vi "Energize.vi"(8 "error in (no error)":errorcluster, 11 "CIFTemplatePlugin in":refnum<class "TemplatePlugin.lvclass">) -> (0 "error out":errorcluster, 3 "CIFTemplatePlugin out":refnum<class "TemplatePlugin.lvclass">)   [LabVIEW 2021, in "TemplatePlugin.lvlib"]
uses:
  TemplatePlugin.lvlib
  Class/TemplatePlugin.lvclass
  D:/dev/CIF-LVCore/src/CIFCore/Class/CIFCorePlugin.lvclass
  CIF-LVCore/src/CIFCore/Class/CIFCorePlugin.lvclass/CIFCorePlugin.ctl
  <vilib>/Platform/TimedLoop/XDataNode/timing_clust.ctl
  <vilib>/Platform/TimedLoop/XDataNode/nitl_modes.ctl
  <vilib>/Platform/TimedLoop/XDataNode/wakeup.ctl
  Class/TemplatePlugin.lvclass/TemplatePlugin.ctl
  CIF-LVCore/src/Channels/CIFChannelMng/CIFChannelMng.lvclass/CIFChannelMng.ctl
  <vilib>/CIF Foundation/CIF Utilities/Statistics/I64/Stats_I64_CIF_U.lvclass/Stats_I64_CIF_U.ctl
  <vilib>/CIF Foundation/CIF Out of Band Commands/CIFOutOfBand.lvclass/CIFOutOfBand.ctl
  CIF-LVCore/src/CIFCore/OOB/OOB_Rx/CIFCoreOOB_Rx.lvclass/CIFCoreOOB_Rx.ctl
  <vilib>/CIF Foundation/CIF Channels Core/CIFChannels/CIFChannels.lvclass/CIFChannels.ctl
  <vilib>/CIF Foundation/CIF Utilities/Time/System Time/Get System Time.vi
  CIF-LVCore/src/CIFCore/Class/SubVIs/Running State Logic.vi
  Class/Dynamic/Execute.vi
  Class/Dynamic/Housekeeping.vi
  CIF-LVCore/src/CIFCore/Class/SubVIs/Send Core OOB TX.vi
  CIF-LVCore/src/CIFCore/Class/Accessors/Read Energized State.vi
  CIF-LVCore/src/CIFCore/Class/SubVIs/Start Running.vi
  <vilib>/CIF Foundation/CIF Utilities/Time/System Time/LabVIEW Time to TAI Time.vi
  CIF-LVCore/src/CIFCore/Class/Accessors/Timestamps/Write Sleep TS.vi
  CIF-LVCore/src/CIFCore/Class/SubVIs/Sleep.vi
  Class/Dynamic/Logic.vi
  CIF-LVCore/src/CIFCore/Class/Accessors/Write Energized State.vi
  CIF-LVCore/src/CIFCore/Class/Benchmarking/Benchmark Running.vi
  CIF-LVCore/src/CIFCore/Class/SubVIs/Read Core OOB RX.vi
  Class/gRPC/Read gRCP to Main.vi
  Class/gRPC/Send Main to gRPC.vi
  CIF-LVCore/src/CIFCore/Class/SubVIs/OOB/Update Status from Benchmarks.vi
  CIF-LVCore/src/Channels/CIFChannelMng/Core/Send Channel List Update.vi
  <vilib>/CIF Foundation/CIF Utilities/Time/System Time/Sleep Until Future Time.vi
  CIF-LVCore/src/CIFCore/Class/Accessors/Timestamps/Write Execute TS.vi
  <vilib>/Utility/error.llb/Clear Errors.vi
  CIF-LVCore/src/CIFCore/Class/Accessors/Read Sleep Limits (ns).vi
  CIF-LVCore/src/CIFCore/Class/Accessors/Timestamps/Write Target Wake TS.vi
  CIF-LVCore/src/CIFCore/Common/Utilities/Add Error.vi
  CIF-LVCore/src/CIFCore/Class/Accessors/Read Plugin Name.vi
  CIF-LVCore/src/CIFCore/Class/Accessors/Timestamps/Read Running TS.vi
  CIF-LVCore/src/CIFCore/Class/Accessors/Read Running Internal Data.vi
  CIF-LVCore/src/CIFCore/Class/Accessors/Read Timing Override.vi
  CIF-LVCore/src/CIFCore/Class/Accessors/Read Common Config.vi
  CIF-LVCore/src/CIFCore/Class/Channel RW/Read Double.vi
  CIF-LVCore/src/CIFCore/Class/Channel RW/Write Double.vi
  CIF-LVCore/src/CIFCore/Class/Channel RW/Read U64.vi
  CIF-LVCore/src/CIFCore/Class/Channel RW/Write U64.vi
  CIF-LVCore/src/CIFCore/Class/Utilities/Benchmarking/Benchmark Custom 1.vi
  Class/Dynamic/Logic.vi/43ad4f59-20dd-452f-bd87-f699ede29eb7.vi
  Class/Dynamic/Logic.vi/a3a5b85b-e031-4b11-917e-7505e820cabf.vi
  CIF-LVCore/src/CIFCore/Class/Accessors/Monitor/Write Double 1.vi
  CIF-LVCore/src/CIFCore/Class/Accessors/Monitor/Write U64 1.vi
  CIF-LVCore/src/CIFCore/Class/Accessors/Monitor/Write I64 1.vi
  CIF-LVCore/src/CIFCore/Class/Accessors/Monitor/Write I64 2.vi
  CIF-LVCore/src/CIFCore/Class/Accessors/Timestamps/Write Housekeeping TS.vi
  <vilib>/CIF Foundation/CIF Utilities/Statistics/I64/X1 minus X0.vi
  <vilib>/CIF Foundation/CIF Utilities/Statistics/I64/Cyclic.vi
  CIF-LVCore/src/CIFCore/Class/Accessors/Timestamps/Read Execute TS.vi
  CIF-LVCore/src/CIFCore/Class/Accessors/Timestamps/Read Housekeeping TS.vi
  CIF-LVCore/src/CIFCore/Class/Accessors/Timestamps/Read Sleep TS.vi
  CIF-LVCore/src/CIFCore/Class/Accessors/Timestamps/Read Target Wake TS.vi
  CIF-LVCore/src/CIFCore/Class/SubVIs/Refresh Stats.vi
  CIF-LVCore/src/CIFCore/OOB/OOB_Rx/Receive/Read Clock Map.vi
  CIF-LVCore/src/Channels/CIFChannelMng/SubVIs/Connect Channel.vi
  CIF-LVCore/src/CIFCore/OOB/OOB_Rx/Receive/Read Connections.vi
  CIF-LVCore/src/CIFCore/OOB/OOB_Rx/Receive/Read Forces.vi
  CIF-LVCore/src/Channels/CIFChannelMng/SubVIs/Force Channel.vi
  CIF-LVCore/src/Channels/CIFChannelMng/SubVIs/Add FIFO Publisher.vi
  CIF-LVCore/src/CIFCore/OOB/OOB_Rx/Receive/Read Publisher Instance.vi
  CIF-LVCore/src/Channels/CIFChannelMng/Core/Send Publisher Instance Return.vi
  CIF-LVCore/src/Channels/CIFChannelMng/SubVIs/Remove FIFO Publisher.vi
  CIF-LVCore/src/CIFCore/OOB/OOB_Rx/Receive/Check for OOB Commands.vi
  OOB/OOB_Rx/Receive/Read Data.vi
  OOB/OOB_Rx/Receive/Check for OOB Commands.vi
  OOB/OOB_Tx/Send/Update Data.vi
  <vilib>/CIF Foundation/CIF Out of Band Commands/Commit Commands.vi
  CIF-LVCore/src/CIFCore/Class/Accessors/Read Refresh.vi
  <vilib>/CIF Foundation/CIF Utilities/Statistics/I64/Get Stats.vi
  CIF-LVCore/src/Channels/CIFChannelMng/OOB/OOB_Tx/Send/Update Channel List Command.vi
  <vilib>/CIF Foundation/CIF Utilities/Time/SubVIs/Add Error.vi
  <vilib>/CIF Foundation/CIF Utilities/Errors/Append Error Location.vi
  CIF-LVCore/src/Channels/CIFChannelMng/Accessors/trash_Read Channel Array.vi
  CIF-LVCore/src/Channels/CIFChannelMng/Accessors/trash_Write Channel Array.vi
  CIF-LVCore/src/CIFCore/Class/Channel RW/Write U64.vi/c8d49817-12f3-40b8-bedc-c305f267c906.vi
  CIF-LVCore/src/CIFCore/Class/Channel RW/Write U64.vi/f151ecc9-1585-4902-b9c5-9b9159353edd.vi
  CIF-LVCore/src/CIFCore/Class/Utilities/Benchmarking/Benchmark Custom 2.vi
  <vilib>/CIF Foundation/CIF Utilities/Statistics/I64/X1 minus X0.vi/dfabcf33-0dbc-4041-80a5-3dc0c86d2989.vi
  <vilib>/CIF Foundation/CIF Utilities/Statistics/I64/Cyclic.vi/dfabcf33-0dbc-4041-80a5-3dc0c86d2989.vi
  CIF-LVCore/src/CIFCore/OOB/OOB_Rx/Private/Read Payload.vi
  CIF-LVCore/src/Channels/CIFChannelMng/Utilities/Get Channel Index by Name.vi
  <vilib>/CIF Foundation/CIF Channels Core/CIFChannels/Accessors/Read Channel State.vi
  <vilib>/CIF Foundation/CIF Channels Core/CIFChannels/Accessors/Read Tag Forced.vi
  CIF-LVCore/src/Channels/CIFChannelMng/SubVIs/Add Error Channel Manager.vi
  CIF-LVCore/src/Channels/CIFChannelMng/OOB/OOB_Tx/Send/FIFO Publisher Return Command.vi
  CIF-LVCore/src/Channels/CIFChannelMng/SubVIs/Get Original FIFO Channel Name.vi
  <vilib>/CIF Foundation/CIF Out of Band Commands/Read Commands.vi
  CIF-LVCore/src/CIFCore/OOB/OOB_Rx/Private/Command Settings.vi
  OOB/OOB_Rx/Private/Read Payload.vi
  OOB/OOB_Rx/Private/Command Settings.vi
  <vilib>/CIF Foundation/CIF Out of Band Commands/Queue Command.vi
  <vilib>/CIF Foundation/CIF Out of Band Commands/Utilities/Command to Bitwise Command.vi
  <vilib>/CIF Foundation/CIF Out of Band Commands/Accessors/Read Local OOB Data.vi
  <vilib>/CIF Foundation/CIF Utilities/Statistics/I64/X1 minus X0.vi/dfabcf33-0dbc-4041-80a5-3dc0c86d2989.vi/9eb60a9a-770f-4d2d-8b3f-8465c267ecc9.vi
  <vilib>/CIF Foundation/CIF Utilities/Statistics/I64/Cyclic.vi/dfabcf33-0dbc-4041-80a5-3dc0c86d2989.vi/9eb60a9a-770f-4d2d-8b3f-8465c267ecc9.vi
  <vilib>/CIF Foundation/CIF Channels Core/ChannelCommon/Utilities/Add Error.vi
  OOB/OOB_Rx/TemplateOOB_Rx.lvclass
  C:/Program Files/National Instruments/LabVIEW 2021/vi.lib/CIF Foundation/CIF Out of Band Commands/CIFOutOfBand.lvclass
  OOB/OOB_Tx/TemplateOOB_Tx.lvclass
  CIF-LVCore/src/Channels/CIFChannelMng/OOB/OOB_Tx/ChnMngOOB_Tx.lvclass
  CIF-LVCore/src/CIFCore/OOB/OOB_Rx/CIFCoreOOB_Rx.lvclass
  CIF-LVCore/src/CIFCore/Class/Logs/Log Run.vi
  <vilib>/CIF Foundation/CIF Channels Core/CIFChannels/Core/Set Force.vi
  <vilib>/Platform/TimedLoop/XDataNode/XDataNode.xnode
  <vilib>/CIF Foundation/CIF Channels Core/CIFChannels/CIFChannels.lvclass
  CIF-LVCore/src/CIFCore/Class/CIFCorePlugin.lvclass
  <vilib>/Platform/TimedLoop/XDataNode/XDNodeRunTimeDep.lvlib
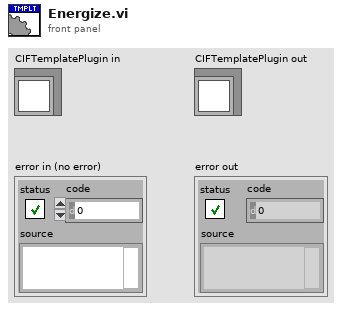
[diagram p1: front panel]
types:
  T1 = typedef "XDNodeRunTimeDep.lvlib/timing_clust.ctl" = cluster{"Expected End [f-1]":u64, "Actual End [f-1]":u64, "Finished Late? [f-1]":bool, "Expected End [i-1]":u64, "Actual End [i-1]":u64, "Finished Late? [i-1]":bool, "Expected Start [i]":u64, "Actual Start [i]":u64, "Expected Start [f]":u64, "Actual Start [f]":u64, "Source Name":string, "Structure Name":string, "Period":i64, "Deadline":i64, "Offset":i64, "Start":i64, "Priority":i32, "Timeout":i32, "Mode":T2, "Wakeup Reason":T3, "Error":errorcluster, "Source Type":string, "Secondary Source Type":string, "Global End Time":u64, "Global Start Time":u64, "Frame Duration":u64, "Iteration Duration":u64, "Assigned CPU":i32, "I/O Scan Engine Mode":u32}
  T2 = typedef "XDNodeRunTimeDep.lvlib/nitl_modes.ctl" = enum32{"No Change", "Process missed periods, maintain original phase", "Discard missed periods, maintain original phase", "Process missed periods, ignore original phase", "Discard missed periods, ignore original phase"}
  T3 = typedef "XDNodeRunTimeDep.lvlib/wakeup.ctl" = enum32{"Normal", "Aborted", "Asynchronous wakeup", "Timing source error", "Timed loop error", "Timeout"}
  T4 = typedef "CIFCorePlugin.lvclass/Prepare State Logic.ctl" = enum16{"Listen", "Prepare", "Error", "Destroy"}
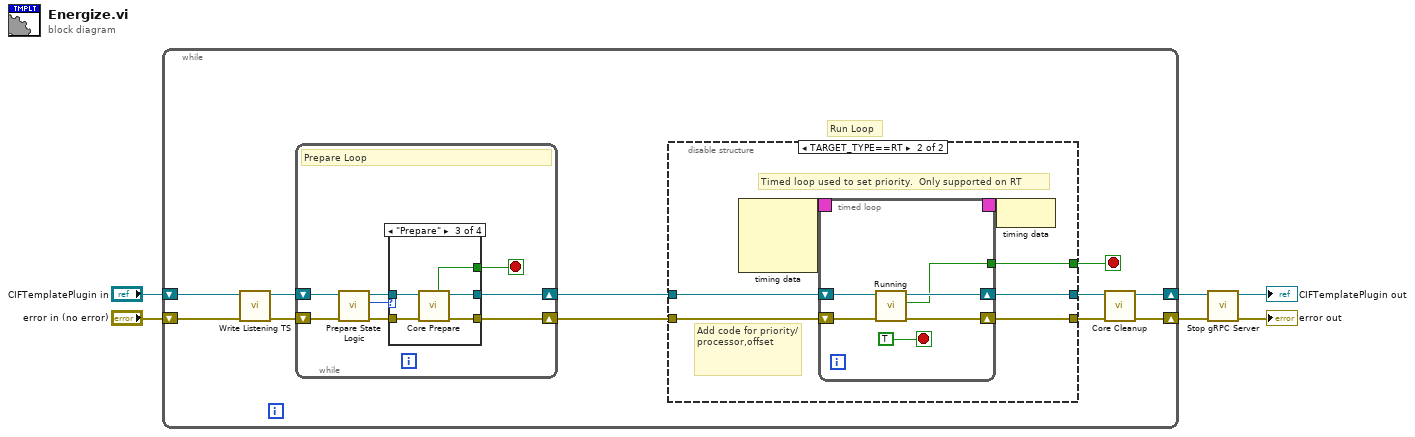
[diagram p0: block diagram]
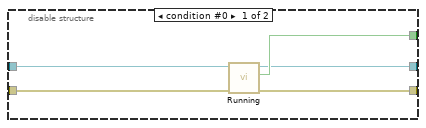
[diagram p2: hidden frame]
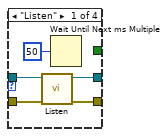
[diagram p3: hidden frame]
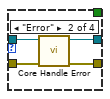
[diagram p4: hidden frame]
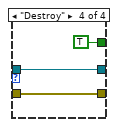
[diagram p5: hidden frame]
diagram:
  n1 = while {
    shift-right: [w14] -> w5
    shift-left: "CIFTemplatePlugin in" -> [w9]
    shift-right: [w13] -> w4
    shift-left: "error in (no error)" -> [w12]
    stop <- w17 stop-if-true
    # "Run Loop"
    n2 = call "Write Listening TS.vi"("error in (no error)"=w12, "CIFCorePlugin in"=w9) -> ("error out"=w10:errorcluster, "CIFCorePlugin out"=w11:refnum<class "TemplatePlugin.lvclass">)  [unwired: 8 in]
    n3 = while {
      shift-right: [w47] -> w8
      shift-left: w11 -> [w40]
      shift-right: [w42] -> w7
      shift-left: w10 -> [w43]
      stop <- w41 stop-if-true
      # "Prepare Loop"
      n4 = call "Prepare State Logic.vi"("error in (no error)"=w43, "CIFCorePlugin in"=w40) -> ("error out"=w44:errorcluster, "Prepare State Logic"=w45:T4, "CIFCorePlugin out"=w46:refnum<class "TemplatePlugin.lvclass">)  [unwired: 7 in]
      n5 = case shown="\"Prepare\"" w45 {
        tunnel: [w48 w56 w61 w64] -> w47
        tunnel: w46 -> [w50 w53 w57 w64]
        tunnel: w44 -> [w51 w54 w58 w63]
        tunnel: [w49 w55 w60 w63] -> w42
        tunnel: [_ _ w59 TRUE ("Transition to Run")] -> w41
        frame "Listen" {
          n6 = call-dynamic "Listen.vi"("error in (no error)"=w51, "CIFTemplatePlugin in"=w50) -> ("error out"=w49:errorcluster, "CIFTemplatePlugin out"=w48:refnum<class "TemplatePlugin.lvclass">)  [unwired: 8 in]
          n7 = Wait Until Next ms Multiple(millisecond multiple=u32 50) -> ()  [unwired: 1 out]
        }
        frame "Error" {
          n8 = call "Core Handle Error.vi"("error in (no error)"=w54, "CIFTemplateNode in"=w53) -> ("error out"=w55:errorcluster, "CIFTemplateNode out"=w56:refnum<class "TemplatePlugin.lvclass">)  [unwired: 8 in]
        }
        frame "Prepare" {
          n9 = call "Core Prepare.vi"("error in (no error)"=w58, "CIFTemplateNode in"=w57) -> ("error out"=w60:errorcluster, "CIFTemplateNode out"=w61:refnum<class "TemplatePlugin.lvclass">, "Transition to Run"=w59:bool)  [unwired: 7 in]
        }
        frame "Destroy" {
        }
      }
    }
    n10 = disable-structure shown="TARGET_TYPE==RT" {
      disable-tunnel: w8 -> [w22 w27]
      disable-tunnel: w7 -> [w21 w26]
      disable-tunnel: [w20 w25] -> w17
      disable-tunnel: [w18 w24] -> w16
      disable-tunnel: [w19 w23] -> w15
      frame condition #0 {
        n11 = call "Running.vi"("error in (no error)"=w21, "CIFTemplatePlugin in"=w22) -> ("error out"=w19:errorcluster, "Destroy"=w20:bool, "CIFTemplatePlugin out"=w18:refnum<class "TemplatePlugin.lvclass">)  [unwired: 7 in]
      }
      frame condition #1 (active) {
        # "Add code for priority/processor,offset"
        # "Timed loop used to set priority.  Only supported on RT"
        n12 = node-c288() -> (w29:T1)  [unwired: 3 in]
        n13 = timed-loop {
          timing: w29 -> [_]
          timing-out: [_] -> w28
          shift-right: [w31] -> w24
          shift-left: w27 -> [w34]
          shift-right: [w32] -> w23
          shift-left: w26 -> [w33]
          tunnel: [w30] -> w25
          stop <- TRUE stop-if-true
          n14 = call "Running.vi"("error in (no error)"=w33, "CIFTemplatePlugin in"=w34) -> ("error out"=w32:errorcluster, "Destroy"=w30:bool, "CIFTemplatePlugin out"=w31:refnum<class "TemplatePlugin.lvclass">)  [unwired: 7 in]
        }
        n15 = node-c288(w28) -> ()
      }
    }
    n16 = call "Core Cleanup.vi"("error in (no error)"=w15, "CIFTemplateNode in"=w16) -> ("error out"=w13:errorcluster, "CIFTemplateNode out"=w14:refnum<class "TemplatePlugin.lvclass">)  [unwired: 8 in]
  }
  n17 = call "Stop gRPC Server.vi"("error in (no error)"=w4, "CIFCorePlugin in"=w5) -> ("error out"=→"error out":errorcluster, "CIFCorePlugin out"=→"CIFTemplatePlugin out":refnum<class "TemplatePlugin.lvclass">)  [unwired: 8 in]
